vi "UpConvert Test Node.vi"(10 "Test Node":T1) -> (2 "Test Node (Extended)":T3)   [LabVIEW 2013, in "Caraya.lvlib" / "Test Result.lvclass"]
uses:
  Test Result.lvclass
  Test Node (Extended).ctl
  Test Registration Data.ctl
  Test Node.ctl
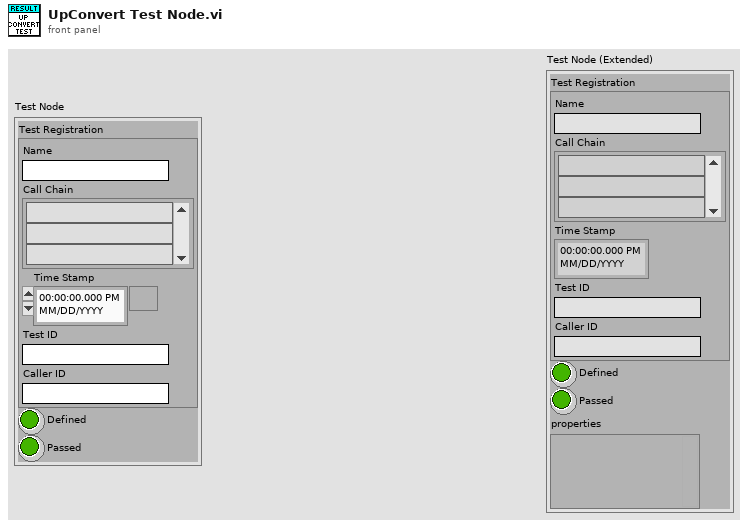
[diagram p1: front panel]
types:
  T1 = typedef "Caraya.lvlib/Test Result.lvclass/Test Node.ctl" = cluster{"Test Registration":T2, "Defined":bool, "Passed":bool}
  T2 = typedef "Caraya.lvlib/Test Result.lvclass/Test Registration Data.ctl" = cluster{"Name":string, "Call Chain":string[], "Time Stamp":timestamp, "Test ID":string, "Caller ID":string}
  T3 = typedef "Caraya.lvlib/Test Result.lvclass/Test Node (Extended).ctl" = cluster{"Test Registration":T2, "Defined":bool, "Passed":bool, "properties":variant}
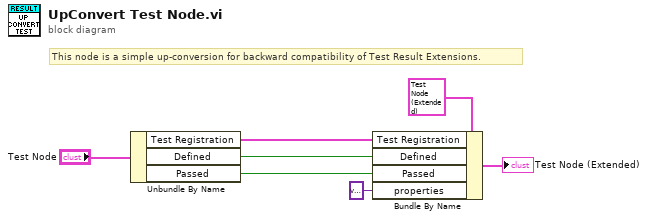
[diagram p0: block diagram]
diagram:
  # "This node is a simple up-conversion for backward compatibility of Test Result Extensions."
  n1 = Unbundle By Name("Test Node") -> ("Test Registration"=w6:T2, "Defined"=w5:bool, "Passed"=w4:bool)
  n2 = Bundle By Name(cluster=T3 {"Test Registration"={"Name"="", "Call Chain"=[], "Time Stamp"=timestamp(0 s since 1904-01-01), "Test ID"="", "Caller ID"=""}, "Defined"=FALSE, "Passed"=FALSE, "properties"=variant} ("Test Node (Extended)"), "Test Registration"=w6, "Defined"=w5, "Passed"=w4, "properties"=variant) -> (→"Test Node (Extended)":T3)
